vi "UpdateUserInterface.vi"(8 "error in (no error)":errorcluster, 10 "DataExchange":T1, 11 "QuickNoteUI in":refnum<class "QuickNoteUI.lvclass">) -> (0 "error out":errorcluster, 2 "DataExchange Out":T1, 3 "QuickNoteUI out":refnum<class "QuickNoteUI.lvclass">)   [LabVIEW 2020, in "QuickNoteUI.lvlib" / "QuickNoteUI.lvclass"]
uses:
  QuickNoteUI.lvclass
  Hardware Abstraction Layer/Component/Device/Device/DataExchange.ctl
  QuickNoteUI.lvclass/QuickNoteUI.ctl
  Hardware Abstraction Layer/Component/GenericActor/GenericActor/GenericController.lvclass
  Interface/DataListener/DataListener.lvclass
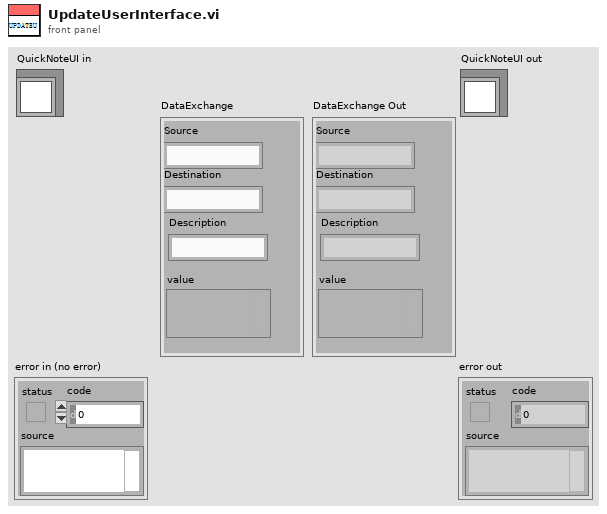
[diagram p1: front panel]
types:
  T1 = typedef "DataListener.lvclass/DataExchange.ctl" = cluster{"Source":string, "Destination":string, "Description":string, "value":variant}
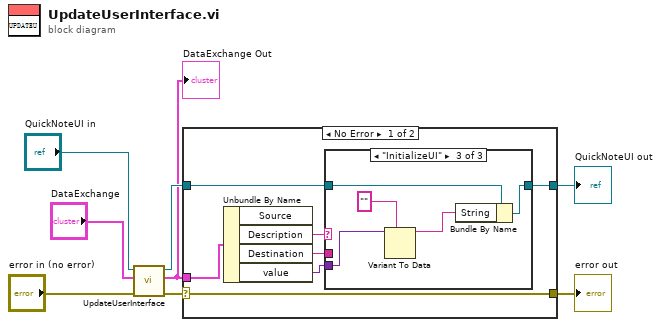
[diagram p0: block diagram]
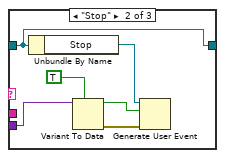
[diagram p3: hidden frame]
diagram:
  n1 = call-parent "UpdateUserInterface.vi"("error in (no error)"="error in (no error)", "DataExchange"="DataExchange", "GenericController in"="QuickNoteUI in") -> ("error out"=w4:errorcluster, "DataExchange Out"=w1:T1, "GenericController out"=w5:refnum<class "QuickNoteUI.lvclass">)  [unwired: 6 in]
  "DataExchange Out" <- w1
  n2 = case shown="No Error" w4 {
    selector: w4 -> [w15 w29]
    tunnel: [w15 w29] -> w2
    tunnel: [w9 w28] -> w3
    tunnel: w5 -> [w10 w28]
    tunnel: w1 -> [w14 _]
    frame No Error {
      n3 = Unbundle By Name(w14) -> ("Description"=w11:string, "Destination"=w12:string, "value"=w13:variant)  [unwired: 1 out]
      n4 = case shown="\"InitializeUI\"" w11 {
        tunnel: w13 -> [_ w22 w27]
        tunnel: w12 -> [_ _ _]
        tunnel: w10 -> [w16 w17 w26]
        tunnel: [w16 w17 w25] -> w9
        frame Default {
        }
        frame "Stop" {
          n5 = Unbundle By Name(w17) -> ("Stop"=w21:refnum<user-event>)
          n6 = Variant To Data(type=TRUE, Variant=w22) -> (data=w20:bool, error out=w18:errorcluster)  [unwired: 1 in]
          n7 = Generate User Event(user event=w21, event data cluster=w20, error in=w18) -> ()  [unwired: 1 in, 2 out]
        }
        frame "InitializeUI" {
          n8 = Variant To Data(type="" ("String"), Variant=w27) -> (data=w23:string)  [unwired: 1 in, 1 out]
          n9 = Bundle By Name(cluster=w26, "String"=w23) -> (w25:refnum<class "QuickNoteUI.lvclass">)
        }
      }
    }
    frame Error {
    }
  }
  "error out" <- w2
  "QuickNoteUI out" <- w3
